vi "Unflatten Header.vi"(7 "offset in":i32, 8 "error in (no error)":errorcluster, 11 "Flattened Data in":u8[](array[numeric])=[0, 0, 0, 0, 0, 0, 0, 0, 0, 0, 0, 0, 0, 0, 0, 0, 0, 0, 0, 0, 0, 0, 0, 0, 0, 0, 0, 0, 0, 0, 0, 0] format="%.0x") -> (0 "error out":errorcluster, 3 "Header out":T1, 5 "offset out":i32)   [LabVIEW 2021, in "ChannelCommon.lvlib"]
uses:
  ChannelCommon.lvlib
  typedef/FIFO Header.ctl
  typedef/Errors.ctl
  <vilib>/CIF Foundation/CIF Utilities/Errors/Append Error Location.vi
  <vilib>/CIF Foundation/CIF Utilities/DataTypes/DataTypes_CIF_U.lvlib
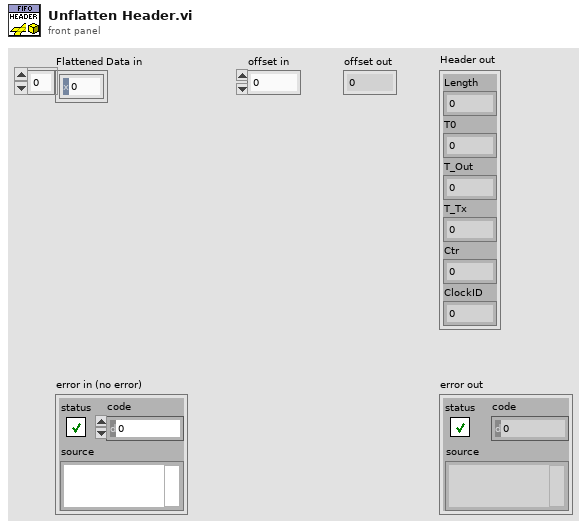
[diagram p1: front panel]
types:
  T1 = typedef "ChannelCommon.lvlib/FIFO Header.ctl" = cluster{"Length":u64, "T0":i64, "T_Out":i64, "T_Tx":i64, "Ctr":u64, "ClockID":u8}
  T2 = typedef "ChannelCommon.lvlib/Errors.ctl" = enum16{"gRPC Server Not Found", "Duplicate Channel", "Missing Channel", "Incorrect Type", "Flatten Error", "Unflatten Data", "Channel Length", "Plugin Connection", "gRPC Server Connection", "FIFO Unflatten"}
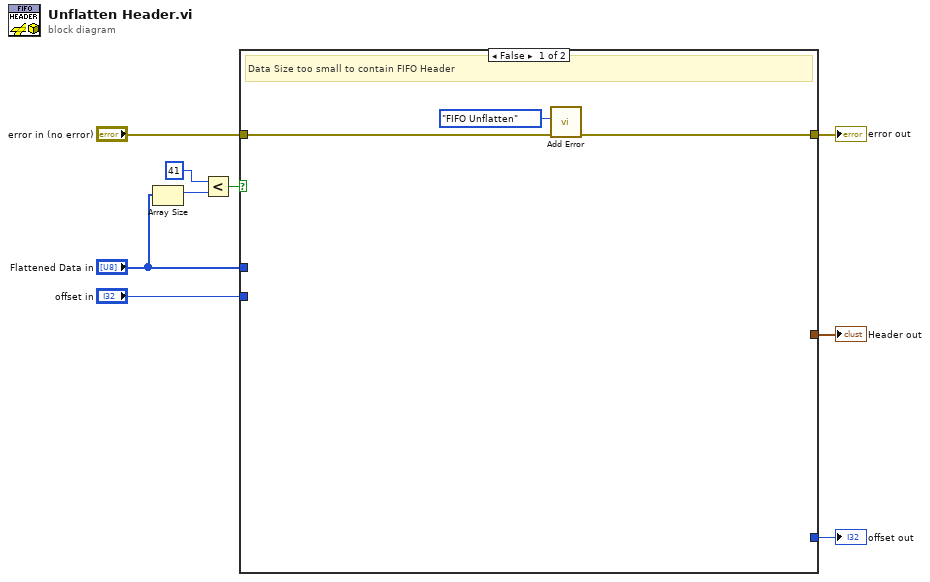
[diagram p0: block diagram]
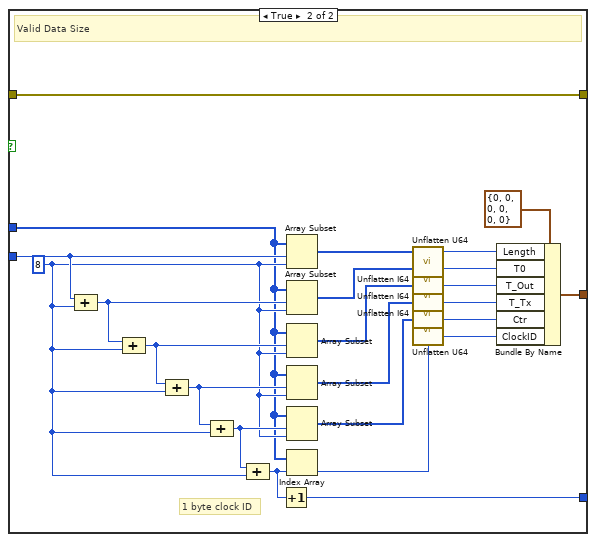
[diagram p2: hidden frame]
diagram:
  n1 = Array Size(array="Flattened Data in") -> (size(s)=w5:i32)
  n2 = Less?(x=41, y=w5) -> (x < y?=w3:bool)
  n3 = case shown="False" w3 {
    tunnel: "offset in" -> [_ w34]
    tunnel: [_ w17] -> w8
    tunnel: [_ w16] -> w7
    tunnel: "Flattened Data in" -> [_ w14]
    tunnel: "error in (no error)" -> [w12 w13]
    tunnel: [w11 w13] -> w1
    frame False {
      # "Data Size too small to contain FIFO Header"
      n4 = call "Add Error.vi"("error in (no error)"=w12, "Error"=Errors."FIFO Unflatten") -> ("error out"=w11:errorcluster)  [unwired: 9 in]
    }
    frame True {
      w18 = 8 ("length")
      # "1 byte clock ID"
      # "Valid Data Size"
      n5 = Compound Arithmetic op=ADD(w34, w18) -> (w33:i32)
      n6 = Compound Arithmetic op=ADD(w33, w18) -> (w32:i32)
      n7 = Compound Arithmetic op=ADD(w32, w18) -> (w31:i32)
      n8 = Compound Arithmetic op=ADD(w31, w18) -> (w27:i32)
      n9 = Compound Arithmetic op=ADD(w27, w18) -> (w26:i32)
      n10 = Increment(x=w26) -> (x+1=w17:i32)
      n11 = Array Subset(array=w14, index=w34, length=w18) -> (w35:u8[])
      n12 = Array Subset(array=w14, index=w33, length=w18) -> (w30:u8[])
      n13 = Array Subset(array=w14, index=w32, length=w18) -> (w29:u8[])
      n14 = Array Subset(array=w14, index=w31, length=w18) -> (w28:u8[])
      n15 = Array Subset(array=w14, index=w27, length=w18) -> (w19:u8[])
      n16 = Index Array(array=w14, index=w26) -> (element=w20:u8)
      n17 = call <vilib>:"Unflatten U64.vi"("Flat Data"=w35) -> ("U64"=w25:u64)  [unwired: 4 in]
      n18 = call <vilib>:"Unflatten I64.vi"("Flat Data"=w30) -> ("I64"=w24:i64)  [unwired: 4 in]
      n19 = call <vilib>:"Unflatten I64.vi"("Flat Data"=w29) -> ("I64"=w23:i64)  [unwired: 4 in]
      n20 = call <vilib>:"Unflatten I64.vi"("Flat Data"=w28) -> ("I64"=w22:i64)  [unwired: 4 in]
      n21 = call <vilib>:"Unflatten U64.vi"("Flat Data"=w19) -> ("U64"=w21:u64)  [unwired: 4 in]
      n22 = Bundle By Name(cluster=T1 {"Length"=0, "T0"=0, "T_Out"=0, "T_Tx"=0, "Ctr"=0, "ClockID"=0} ("Header in"), "Length"=w25, "T0"=w24, "T_Out"=w23, "T_Tx"=w22, "Ctr"=w21, "ClockID"=w20) -> (w16:T1)
    }
  }
  "Header out" <- w7
  "offset out" <- w8
  "error out" <- w1
